vi "lvBuild.vi"   [LabVIEW 2014, in "G CLI LvBuild.lvlib"]
uses:
  G CLI LvBuild.lvlib
  <vilib>/Wiresmith Technology/G CLI/Argument Parser/Option Class/Option Configuration.ctl
  <vilib>/Wiresmith Technology/G CLI/Argument Parser/Option Class/Argument Type.ctl
  <vilib>/AppBuilder/AB_API_Simple/Build (path).vi
  <vilib>/Wiresmith Technology/G CLI/CLI Class/CLI.lvclass
  <vilib>/Wiresmith Technology/G CLI/Argument Parser/Option Set Class/Option Set.lvclass
  <vilib>/Wiresmith Technology/G CLI/Argument Parser/Option Class/Option.lvclass
  <vilib>/AppBuilder/AB_API_Simple/NI_App_Builder_API.lvlib
types:
  T1 = typedef "Option Parser.lvlib/Option.lvclass/Option Configuration.ctl" = cluster{"Option Type":T2, "Option Labels":string[], "Key":string, "Description":string, "Required":bool, "Default Value":string}
  T2 = typedef "Option Parser.lvlib/Option.lvclass/Argument Type.ctl" = enum16{"flag", "value"}
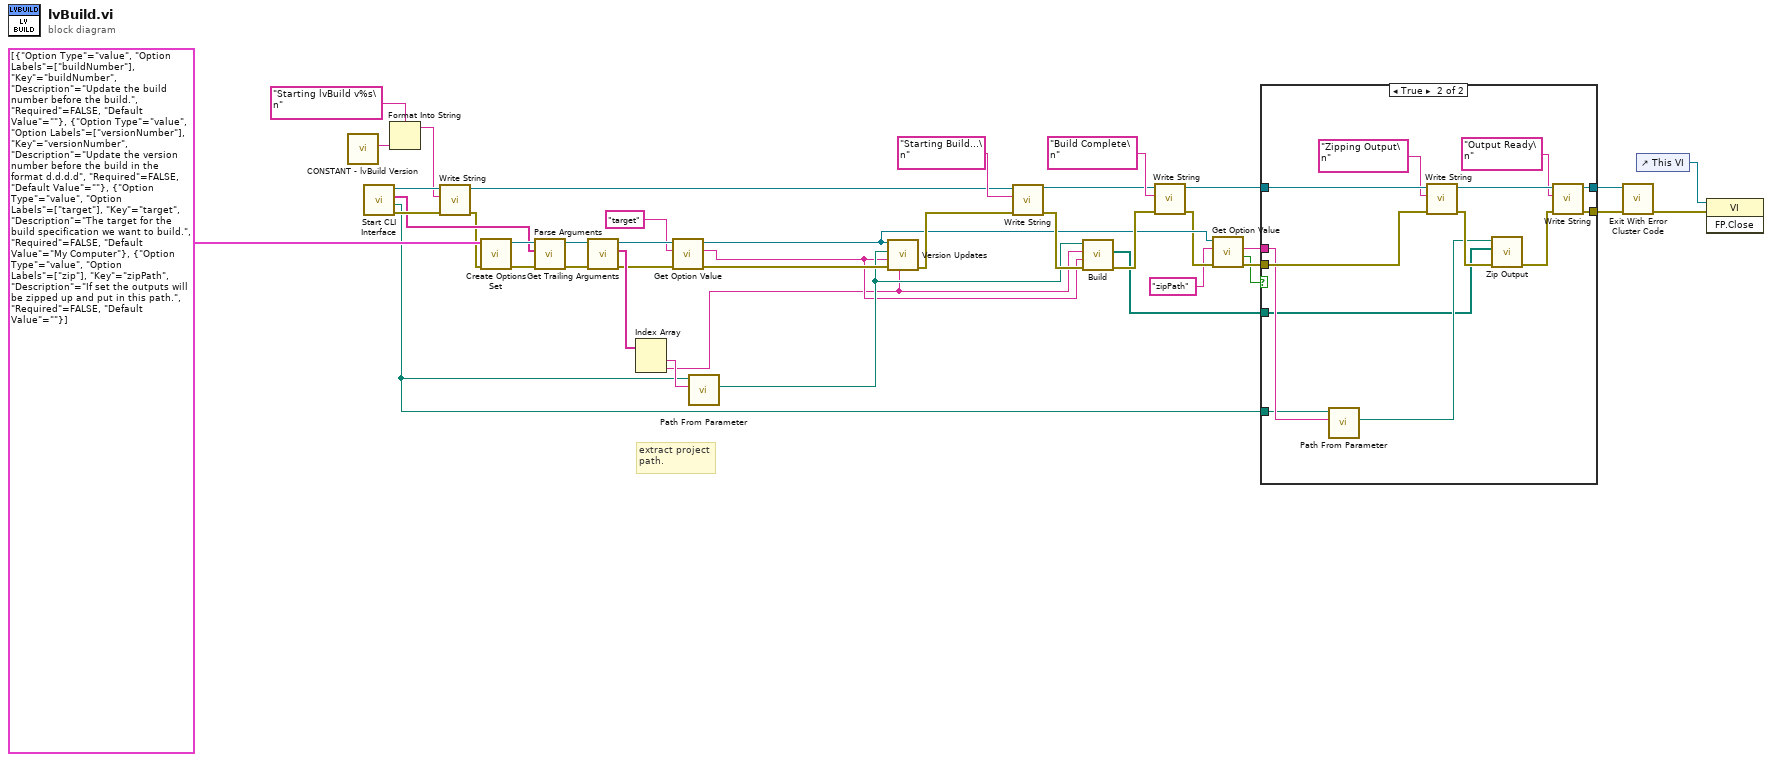
[diagram p0: block diagram]
diagram:
  # "extract project\npath."
  n1 = call "CONSTANT - lvBuild Version.vi"() -> ("Version"=w13:string)  [unwired: 11 in]
  n2 = call <vilib>:"Start CLI Interface.vi"() -> ("error out"=w39:errorcluster, "Working Directory"=w2:path, "Custom Parameters"=w36:string[], "CLI out"=w17:refnum<class "CLI.lvclass">)  [unwired: 8 in]
  n3 = Format Into String(format string="Starting lvBuild v%s\n", w13) -> (resulting string=w14:string)  [unwired: 2 in, 1 out]
  n4 = call <vilib>:"Write String.vi"("error in (no error)"=w39, "Text to Write"=w14, "CLI in"=w17) -> ("error out"=w18:errorcluster, "CLI out"=w16:refnum<class "CLI.lvclass">)  [unwired: 7 in]
  n5 = call <vilib>:"Create Options Set.vi"("error in (no error)"=w18, "Options"=T1[] [{"Option Type"=enum."value", "Option Labels"=["buildNumber"], "Key"="buildNumber", "Description"="Update the build number before the build.", "Required"=FALSE, "Default Value"=""}, {"Option Type"=enum."value", "Option Labels"=["versionNumber"], "Key"="versionNumber", "Description"="Update the version number before the build in the format d.d.d.d", "Required"=FALSE, "Default Value"=""}, {"Option Type"=enum."value", "Option Labels"=["target"], "Key"="target", "Description"="The target for the build specification we want to build.", "Required"=FALSE, "Default Value"="My Computer"}, {"Option Type"=enum."value", "Option Labels"=["zip"], "Key"="zipPath", "Description"="If set the outputs will be zipped up and put in this path.", "Required"=FALSE, "Default Value"=""}]) -> ("error out"=w37:errorcluster, "Option Set out"=w38:refnum<class "Option Set.lvclass">)  [unwired: 8 in]
  n6 = call <vilib>:"Parse Arguments.vi"("error in (no error)"=w37, "Arguments"=w36, "Option Set in"=w38) -> ("error out"=w34:errorcluster, "Option Set out"=w35:refnum<class "Option Set.lvclass">)  [unwired: 5 in, 2 out]
  n7 = call <vilib>:"Get Trailing Arguments.vi"("error in (no error)"=w34, "Option Set in"=w35) -> ("error out"=w31:errorcluster, "Arguments"=w33:string[], "Option Set out"=w29:refnum<class "Option Set.lvclass">)  [unwired: 7 in]
  n8 = Index Array(array=w33) -> (element #1=w32:string, element #2=w20:string)  [unwired: 2 in]
  n9 = call <vilib>:"Get Option Value.vi"("error in (no error)"=w31, "Option Key"="target", "Option Set in"=w29) -> ("error out"=w30:errorcluster, "Value"=w21:string, "Option Set out"=w10:refnum<class "Option Set.lvclass">)  [unwired: 5 in, 1 out]
  n10 = call <vilib>:"Path From Parameter.vi"("Path Parameter"=w32, "Working Directory"=w2) -> ("Full Path"=w22:path)  [unwired: 9 in]
  n11 = call "Version Updates.vi"("Build Spec"=w20, "error in (no error)"=w30, "Target"=w21, "Project"=w22, "Option Set in"=w10) -> ("error out"=w27:errorcluster)  [unwired: 6 in]
  n12 = call <vilib>:"Write String.vi"("error in (no error)"=w27, "Text to Write"="Starting Build...\n", "CLI in"=w16) -> ("error out"=w25:errorcluster, "CLI out"=w19:refnum<class "CLI.lvclass">)  [unwired: 7 in]
  n13 = call-poly <vilib>:"Build.vi"("error in (no error)"=w25, "Name of target (My Computer)"=w21, "Name of build specification (if empty: build all)"=w20, "Path to project"=w22) -> ("error out"=w26:errorcluster, "Generated files"=w1:path[])  [unwired: 6 in]
  n14 = call <vilib>:"Write String.vi"("error in (no error)"=w26, "Text to Write"="Build Complete\n", "CLI in"=w19) -> ("error out"=w9:errorcluster, "CLI out"=w41:refnum<class "CLI.lvclass">)  [unwired: 7 in]
  n15 = call <vilib>:"Get Option Value.vi"("error in (no error)"=w9, "Option Key"="zipPath", "Option Set in"=w10) -> ("error out"=w6:errorcluster, "Set"=w4:bool, "Value"=w3:string)  [unwired: 5 in, 1 out]
  n16 = case shown="True" w4 {
    tunnel: w41 -> [w43 w56]
    tunnel: [w43 w54] -> w8
    tunnel: [w42 w53] -> w7
    tunnel: w6 -> [w42 w50]
    tunnel: w3 -> [_ w47]
    tunnel: w2 -> [_ w46]
    tunnel: w1 -> [_ w44]
    frame False {
    }
    frame True {
      n17 = call <vilib>:"Path From Parameter.vi"("Path Parameter"=w47, "Working Directory"=w46) -> ("Full Path"=w45:path)  [unwired: 9 in]
      n18 = call <vilib>:"Write String.vi"("error in (no error)"=w50, "Text to Write"="Zipping Output\n", "CLI in"=w56) -> ("error out"=w51:errorcluster, "CLI out"=w55:refnum<class "CLI.lvclass">)  [unwired: 7 in]
      n19 = call "Zip Output.vi"("error in (no error)"=w51, "Generated Files"=w44, "Zip File Location"=w45) -> ("error out"=w52:errorcluster)  [unwired: 8 in]
      n20 = call <vilib>:"Write String.vi"("error in (no error)"=w52, "Text to Write"="Output Ready\n", "CLI in"=w55) -> ("error out"=w53:errorcluster, "CLI out"=w54:refnum<class "CLI.lvclass">)  [unwired: 7 in]
    }
  }
  n21 = call <vilib>:"Exit With Error Cluster Code.vi"("error in (no error)"=w7, "CLI in"=w8) -> ("error out"=w11:errorcluster)  [unwired: 9 in]
  n22 = control-ref of="This VI"() -> (w12:refnum<vi>)
  n23 = invoke class="VI" method="FP.Close"(reference=w12, error in=w11) -> ()  [unwired: 1 in, 3 out]
